vi "Test Worker Waiting After Completing Job.vi"(8 "error in (no error)":errorcluster, 11 "Worker Test in":refnum<class "Worker Test.lvclass">) -> (0 "error out":errorcluster, 3 "Worker Test out":refnum<class "Worker Test.lvclass">)   [LabVIEW 2020, in "Worker Test.lvclass"]
uses:
  Worker Test.lvclass
  C:/Program Files (x86)/National Instruments/LabVIEW 2020/vi.lib/Asteme/LUnit/Test Case.lvclass
  Test Doubles/Stub Job Handler/Stub Job Handler.lvclass
  C:/Users/anton/Documents/GitHub/Triarc-Examples/Coffee Shop/Process Job/Job Handler.lvclass
  <vilib>/Asteme/Triarc Framework/Process/Process.lvclass/Process.ctl
  <vilib>/Asteme/LUnit/Test Case.lvclass/Test Case.ctl
  <vilib>/Asteme/LUnit/LUnit Assertion Result.lvclass/LUnit Assertion Result.ctl
  <vilib>/Asteme/Triarc Framework Test Suite/Support/Execution timer.vi
  <vilib>/Asteme/Triarc Framework/Process/Private/SubVIs/Wait for finish.vi
  <vilib>/Asteme/Triarc Framework/Process/Protected/Messaging/Enqueue Message.vi
  <vilib>/Asteme/Triarc Framework/Process/Private/SubVIs/Set Lifecycle State.vi
  <vilib>/Asteme/Triarc Framework/Process/Public/Lifecycle/Get Lifecycle State.vi
  <vilib>/Asteme/LUnit/Palette/Pass If.vi
  <vilib>/Asteme/LUnit/Set Assertion Type.vi
  <vilib>/AdvancedString/1D String Array to Delimited String.vi
  <vilib>/Utility/error.llb/Clear Errors.vi
  <vilib>/Asteme/LUnit/Palette/Fail.vi
  <vilib>/Asteme/LUnit/Palette/Pass.vi
  <vilib>/Asteme/LUnit/LUnit Write Assertion Type.vi
  <vilib>/Asteme/LUnit/Add test result.vi
  <vilib>/Asteme/LUnit/LUnit Write Passed.vi
  <vilib>/Asteme/LUnit/LUnit Get Test Case.vi
  <vilib>/Asteme/LUnit/Assertion Result/LUnit Get Test Name.vi
  <vilib>/Asteme/LUnit/LUnit Write Message.vi
  <vilib>/Asteme/LUnit/LUnit Write Description.vi
  <vilib>/Asteme/LUnit/Read Test Case Name.vi
  Processes/People/Workers/Worker/Worker.lvclass
  C:/Program Files (x86)/National Instruments/LabVIEW 2020/vi.lib/Asteme/Triarc Framework/Process/Process.lvclass
  <vilib>/Asteme/Triarc Framework Test Suite/Support/Event Helpers/Dequeue Event Message.vi
  <vilib>/Utility/error.llb/Error Cluster From Error Code.vi
  <vilib>/Asteme/LUnit/LUnit Assertion Result.lvclass
  <vilib>/Asteme/Triarc Framework/Process/Process.lvclass
  <vilib>/Asteme/Triarc Framework Test Suite/Support/Event Helpers/Event Helpers.lvlib
  <vilib>/Asteme/LUnit/Test Case.lvclass
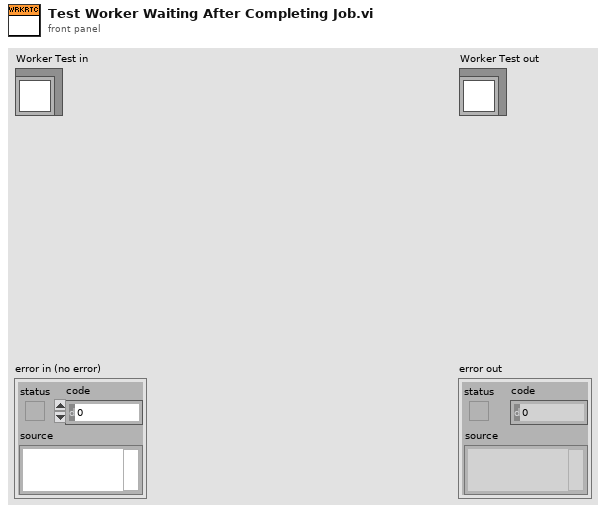
[diagram p1: front panel]
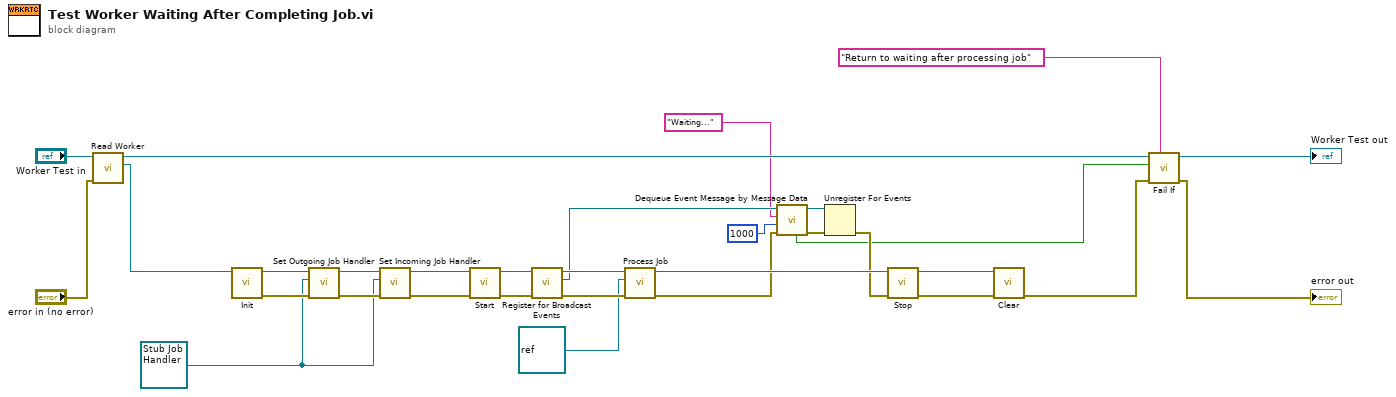
[diagram p0: block diagram]
diagram:
  w1 = refnum<class "Stub Job Handler.lvclass"> refnum ("Stub Job Processor.lvclass")
  n1 = call "Read Worker.vi"("error in (no error)"="error in (no error)", "Worker Test in"="Worker Test in") -> ("Worker"=w26:refnum<class "Worker.lvclass">, "Worker Test out"=w28:refnum<class "Worker Test.lvclass">)  [unwired: 7 in, 1 out]
  n2 = call-dynamic "Init.vi"("View In"=w26) -> ("error out"=w6:errorcluster, "View Out"=w7:refnum<class "Worker.lvclass">)  [unwired: 9 in]
  n3 = call "Set Outgoing Job Handler.vi"("error in (no error)"=w6, "Work Dispatcher"=w1, "Worker In"=w7) -> ("error out"=w2:errorcluster, "Worker Out"=w5:refnum<class "Worker.lvclass">)  [unwired: 7 in]
  n4 = call "Set Incoming Job Handler.vi"("error in (no error)"=w2, "Job Handler"=w1, "Worker In"=w5) -> ("error out"=w3:errorcluster, "Worker Out"=w4:refnum<class "Worker.lvclass">)  [unwired: 7 in]
  n5 = call <vilib>:"Start.vi"("error in (no error)"=w3, "Process In"=w4) -> ("error out"=w23:errorcluster, "Process Out"=w19:refnum<class "Worker.lvclass">)  [unwired: 8 in]
  n6 = call <vilib>:"Register for Broadcast Events.vi"("error in (no error)"=w23, "Process In"=w19) -> ("error out"=w20:errorcluster, "Event Registration Refnum Out"=w14:refnum<event-registration>, "Process Out"=w18:refnum<class "Worker.lvclass">)  [unwired: 7 in]
  n7 = call-dynamic "Process Job.vi"("error in (no error)"=w20, "Job"=refnum<class> refnum ("Task"), "Worker In"=w18) -> ("error out"=w16:errorcluster, "Worker Out"=w17:refnum<class "Worker.lvclass">)  [unwired: 7 in]
  n8 = call <vilib>:"Dequeue Event Message by Message Data.vi"("error in (no error)"=w16, "Timeout (-1)"=1000, "Message Data"="Waiting...", "Event Registration Refnum"=w14) -> ("error out"=w11:errorcluster, "Event Registration Refnum Out"=w9:refnum<event-registration>, "Timed Out?"=w8:bool)  [unwired: 3 in, 2 out]
  n9 = Unregister For Events(event registration refnum=w9, error in=w11) -> (error out=w10:errorcluster)
  n10 = call <vilib>:"Stop.vi"("error in (no error)"=w10, "Process In"=w17) -> ("error out"=w24:errorcluster, "Process Out"=w25:refnum<class "Worker.lvclass">)  [unwired: 7 in, 1 out]
  n11 = call-dynamic "Clear.vi"("error in (no error)"=w24, "View In"=w25) -> ("error out"=w22:errorcluster)  [unwired: 9 in]
  n12 = call <vilib>:"Fail If.vi"("Description"="Return to waiting after processing job", "error in (no error)"=w22, "Fail?"=w8, "Test Case In"=w28) -> ("error out"=→"error out":errorcluster, "Test Case Out"=→"Worker Test out":refnum<class "Worker Test.lvclass">)  [unwired: 6 in]
